vi "test1-ResponseWithError.vi"(8 "error in (no error)":errorcluster, 11 "TestCase in":refnum<class "testcase-CSMResponse.lvclass">) -> (0 "error out":errorcluster, 3 "TestCase out":refnum<class "testcase-CSMResponse.lvclass">)   [LabVIEW 2017, in "testcase-CSMResponse.lvclass"]
uses:
  testcase-CSMResponse.lvclass
  68a58439-6a05-4de0-8ad5-cfc0558cbd3a.vi
  <vilib>/addons/_JKI Toolkits/VI Tester/TestCase.llb/TestCase.lvclass
  src/user.lib/_NEVSTOP/Communicable State Machine(CSM)/Communicable State Machine.lvlib
  CSM/CSM-Testcase.lvlib
  C:/Program Files (x86)/National Instruments/LabVIEW 2017/vi.lib/addons/_JKI Toolkits/VI Tester/TestCase.llb/TestCase.lvclass
panel:
  out "Loopcount":i32
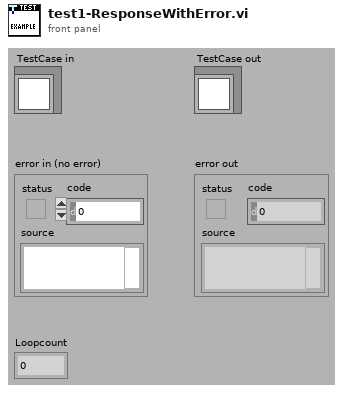
[diagram p1: front panel]
types:
  T1 = cluster{"Arguments":string, "Response":string, "error":errorcluster}
  T2 = cluster{"status":bool, "code":bool, "source":bool}
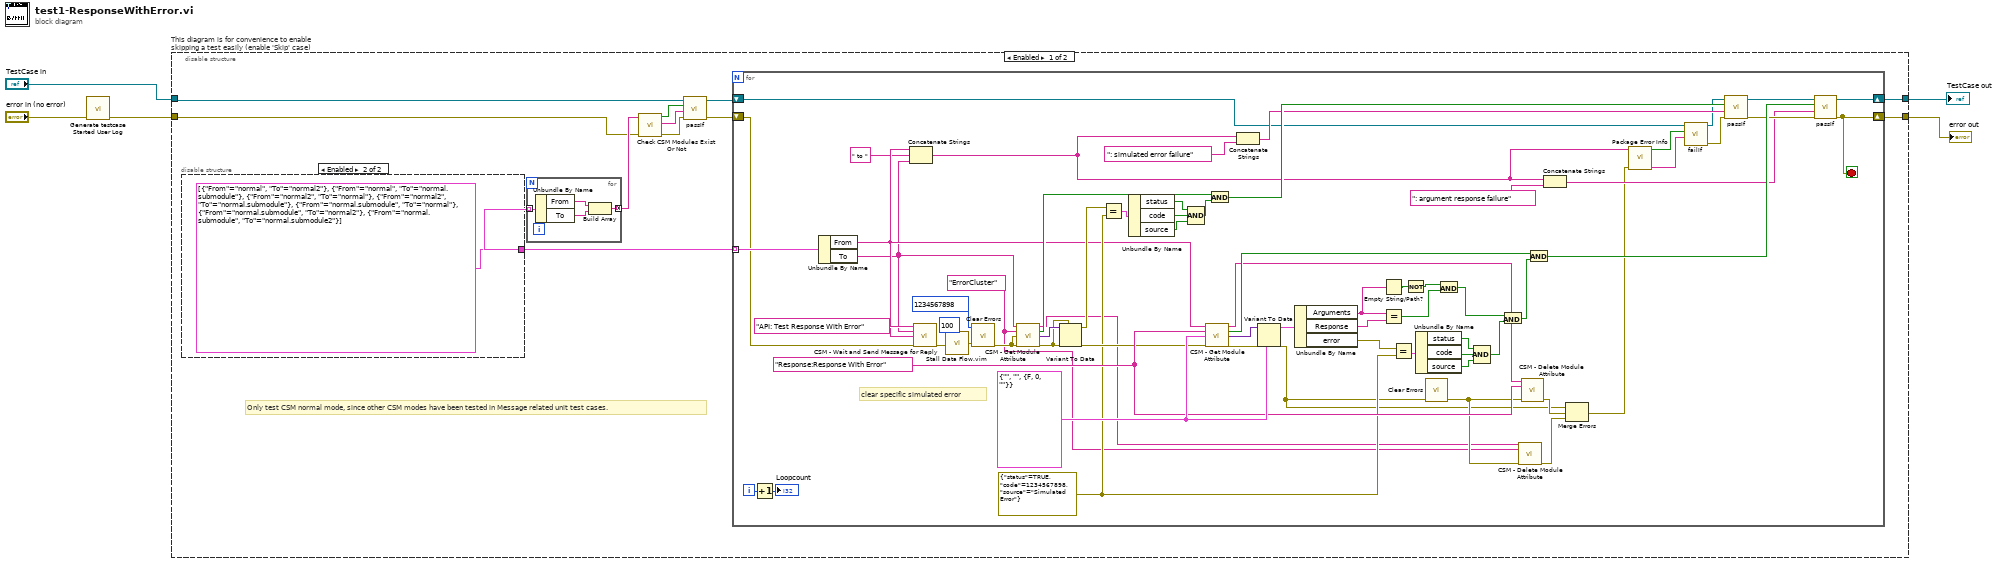
[diagram p0: block diagram]
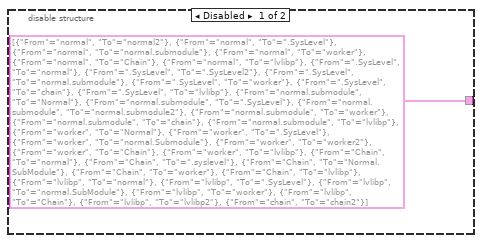
[diagram p2: hidden frame]
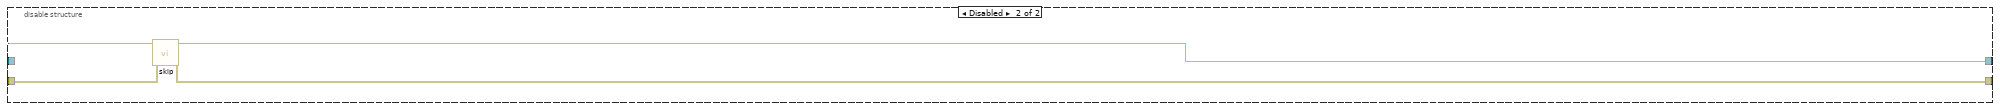
[diagram p3: hidden frame]
diagram:
  n1 = call "Generate testcase Started User Log.vi"("Error In"="error in (no error)") -> ("error out"=w1:errorcluster)  [unwired: 10 in]
  n2 = disable-structure "This diagram is for convenience to enable skipping a test easily (enable 'Skip' case)" shown="Enabled" {
    disable-tunnel: "TestCase in" -> [w10 w93]
    disable-tunnel: [w16 w91] -> w2
    disable-tunnel: [w15 w92] -> w4
    disable-tunnel: w1 -> [w7 w90]
    frame Enabled {
      # "Only test CSM normal mode, since other CSM modes have been tested in Message related unit test cases."
      n3 = disable-structure shown="Enabled" {
        disable-tunnel: [cluster{"From":string, "To":string}[] [{"From"="normal", "To"="normal2"}, {"From"="normal", "To"=".SysLevel"}, {"From"="normal", "To"="normal.submodule"}, {"From"="normal", "To"="worker"}, {"From"="normal", "To"="Chain"}, {"From"="normal", "To"="lvlibp"}, {"From"=".SysLevel", "To"="normal"}, {"From"=".SysLevel", "To"=".SysLevel2"}, {"From"=".SysLevel", "To"="normal.submodule"}, {"From"=".SysLevel", "To"="worker"}, {"From"=".SysLevel", "To"="chain"}, {"From"=".SysLevel", "To"="lvlibp"}, {"From"="normal.submodule", "To"="Normal"}, {"From"="normal.submodule", "To"=".SysLevel"}, {"From"="normal.submodule", "To"="normal.submodule2"}, {"From"="normal.submodule", "To"="worker"}, {"From"="normal.submodule", "To"="chain"}, {"From"="normal.submodule", "To"="lvlibp"}, {"From"="worker", "To"="Normal"}, {"From"="worker", "To"=".SysLevel"}, {"From"="worker", "To"="normal.Submodule"}, {"From"="worker", "To"="worker2"}, {"From"="worker", "To"="Chain"}, {"From"="worker", "To"="lvlibp"}, {"From"="Chain", "To"="normal"}, {"From"="Chain", "To"=".syslevel"}, {"From"="Chain", "To"="Normal.SubModule"}, {"From"="Chain", "To"="worker"}, {"From"="Chain", "To"="lvlibp"}, {"From"="lvlibp", "To"="normal"}, {"From"="lvlibp", "To"=".SysLevel"}, {"From"="lvlibp", "To"="normal.SubModule"}, {"From"="lvlibp", "To"="worker"}, {"From"="lvlibp", "To"="Chain"}, {"From"="lvlibp", "To"="lvlibp2"}, {"From"="chain", "To"="chain2"}] cluster{"From":string, "To":string}[] [{"From"="normal", "To"="normal2"}, {"From"="normal", "To"="normal.submodule"}, {"From"="normal2", "To"="normal"}, {"From"="normal2", "To"="normal.submodule"}, {"From"="normal.submodule", "To"="normal"}, {"From"="normal.submodule", "To"="normal2"}, {"From"="normal.submodule", "To"="normal.submodule2"}]] -> w6
        frame Disabled {
        }
        frame Enabled {
        }
      }
      n4 = for {
        tunnel: w6 -> [w22] mode=indexing
        tunnel: [w19] -> w13 mode=concatenating
        n5 = Unbundle By Name(w22) -> ("From"=w21:string, "To"=w20:string)
        n6 = Build Array(w21, w20) -> (w19:string[])
      }
      n7 = call "Check CSM Modules Exist Or Not.vi"("error in"=w7, "CSM names in"=w13) -> ("error out"=w11:errorcluster, "Debug string"=w12:string, "All Modules Exist?"=w14:bool)  [unwired: 7 in]
      n8 = call-dynamic "passIf.vi"("error in (no error)"=w11, "message (\"\")"=w12, "pass"=w14, "TestCase in"=w10) -> ("error out"=w8:errorcluster, "TestCase out"=w9:refnum<class "testcase-CSMResponse.lvclass">)  [unwired: 6 in]
      n9 = for {
        tunnel: w6 -> [w80] mode=indexing
        shift-right: [w89] -> w16
        shift-left: w9 -> [w28]
        shift-right: [w31] -> w15
        shift-left: w8 -> [w42]
        i -> [w65]
        stop <- w31 stop-if-true
        w43 = "ErrorCluster" ("Attribute")
        w54 = errorcluster {"status"=TRUE, "code"=1234567898, "source"="Simulated Error"} ("error out")
        w86 = T1 {"Arguments"="", "Response"="", "error"={"status"=FALSE, "code"=0, "source"=""}}
        w78 = "Response:Response With Error" ("State")
        # "clear specific simulated error"
        n10 = Increment(x=w65) -> (x+1=→"Loopcount":i32)
        n11 = Unbundle By Name(w80) -> ("From"=w38:string, "To"=w37:string)
        n12 = Concatenate Strings(w38, " to " ("string"), w37) -> (w23:string)
        n13 = call "CSM - Wait and Send Message for Reply.vi"("State"="API: Test Response With Error", "Arguments (\"\")"=w37, "Target Module"=w38, "Error In (No Error)"=w42) -> ("error out"=w63:errorcluster)  [unwired: 8 in, 3 out]
        n14 = call "Stall Data Flow.vim"("value in"=w63, "milliseconds to wait"=u32 100) -> ("value out"=w62:errorcluster)  [unwired: 1 out]
        n15 = call <vilib>:"Clear Errors.vi"("error in (no error)"=w62, "specific error code to clear (0: all)"=1234567898) -> ("error out"=w60:errorcluster)  [unwired: 4 in, 1 out]
        n16 = call "CSM - Get Module Attribute.vi"("CSM Name"=w37, "Attribute"=w43, "Default Value (Empty Variant)"=w60, "Error In"=w60) -> ("CSM Name (Dup)"=w44:string, "Found"=w59:bool, "Value"=w57:variant, "error out"=w56:errorcluster)  [unwired: 7 in, 1 out]
        n17 = Variant To Data(error in=w56, type=w56, Variant=w57) -> (data=w55:errorcluster, error out=w58:errorcluster)
        n18 = Equal?(x=w55, y=w54) -> (x = y?=w50:T2)
        n19 = Unbundle By Name(w50) -> ("status"=w51:bool, "code"=w52:bool, "source"=w53:bool)
        n20 = Compound Arithmetic op=AND(w51, w52, w53) -> (w49:bool)
        n21 = call "CSM - Get Module Attribute.vi"("CSM Name"=w38, "Attribute"=w78, "Default Value (Empty Variant)"=w86, "Error In"=w58) -> ("CSM Name (Dup)"=w79:string, "Found"=w83:bool, "Value"=w85:variant, "error out"=w87:errorcluster)  [unwired: 7 in, 1 out]
        n22 = And(x=w59, y=w49) -> (x .and. y?=w48:bool)
        n23 = Concatenate Strings(w23, ": simulated error failure" ("string")) -> (w34:string)
        n24 = Variant To Data(error in=w87, type=w86, Variant=w85) -> (data=w84:T1, error out=w39:errorcluster)
        n25 = Unbundle By Name(w84) -> ("Arguments"=w73:string, "Response"=w72:string, "error"=w71:errorcluster)
        n26 = Empty String/Path?(string/path=w73) -> (empty?=w77:bool)
        n27 = Equal?(x=w73, y=w72) -> (x = y?=w75:bool)
        n28 = Equal?(x=w71, y=w54) -> (x = y?=w70:T2)
        n29 = Not(x=w77) -> (.not. x?=w76:bool)
        n30 = Unbundle By Name(w70) -> ("status"=w69:bool, "code"=w68:bool, "source"=w67:bool)
        n31 = call <vilib>:"Clear Errors.vi"("error in (no error)"=w39) -> ("error out"=w45:errorcluster)  [unwired: 5 in, 1 out]
        n32 = And(x=w76, y=w75) -> (x .and. y?=w74:bool)
        n33 = Compound Arithmetic op=AND(w69, w68, w67) -> (w66:bool)
        n34 = And(x=w74, y=w66) -> (x .and. y?=w82:bool)
        n35 = call "CSM - Delete Module Attribute.vi"("CSM Name"=w44, "Attribute"=w43, "Error In"=w45) -> ("error out"=w25:errorcluster)  [unwired: 9 in, 3 out]
        n36 = call "CSM - Delete Module Attribute.vi"("CSM Name"=w79, "Attribute"=w78, "Error In"=w45) -> ("error out"=w40:errorcluster)  [unwired: 9 in, 3 out]
        n37 = And(x=w83, y=w82) -> (x .and. y?=w81:bool)
        n38 = Concatenate Strings(w23, ": argument response failure" ("string")) -> (w32:string)
        n39 = Merge Errors(w39, w40, w25) -> (w24:errorcluster)
        n40 = call "Package Error Info.vi"("error in"=w24, "String in"=w23) -> ("packed error info out"=w29:string, "error status"=w30:bool)  [unwired: 8 in]
        n41 = call-dynamic "failIf.vi"("message (\"\")"=w29, "fail"=w30, "TestCase in"=w28) -> ("error out"=w26:errorcluster, "TestCase out"=w27:refnum<class "testcase-CSMResponse.lvclass">)  [unwired: 7 in]
        n42 = call-dynamic "passIf.vi"("error in (no error)"=w26, "message (\"\")"=w34, "pass"=w48, "TestCase in"=w27) -> ("error out"=w47:errorcluster, "TestCase out"=w46:refnum<class "testcase-CSMResponse.lvclass">)  [unwired: 6 in]
        n43 = call-dynamic "passIf.vi"("error in (no error)"=w47, "message (\"\")"=w32, "pass"=w81, "TestCase in"=w46) -> ("error out"=w31:errorcluster, "TestCase out"=w89:refnum<class "testcase-CSMResponse.lvclass">)  [unwired: 6 in]
      }
    }
    frame Disabled {
      # "skip test result while test is under development"
      n44 = call <vilib>:"skip.vi"("error in (no error)"=w90, "TestCase in"=w93) -> ("error out"=w92:errorcluster, "TestCase out"=w91:refnum<class "testcase-CSMResponse.lvclass">)  [unwired: 8 in]
    }
  }
  "error out" <- w4
  "TestCase out" <- w2
